vi "Set Window Topmost--lvapt.vi"(6 "Topmost(T)/Normal(F)":bool=TRUE, 8 "error in (no error)":errorcluster) -> (0 "error out":errorcluster)   [LabVIEW 2019]
uses:
  de497024-60f2-4a57-aa28-fde8f66e810e.vi
  WINUTIL.LLB/WINUTIL.lvlib
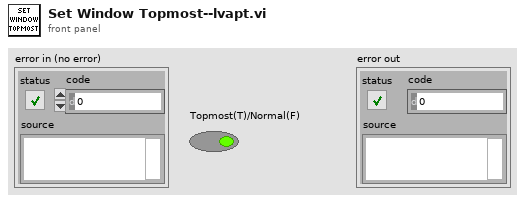
[diagram p1: front panel]
types:
  T1 = typedef "WINUTIL.lvlib/Window Refnum" = refnum<k1>
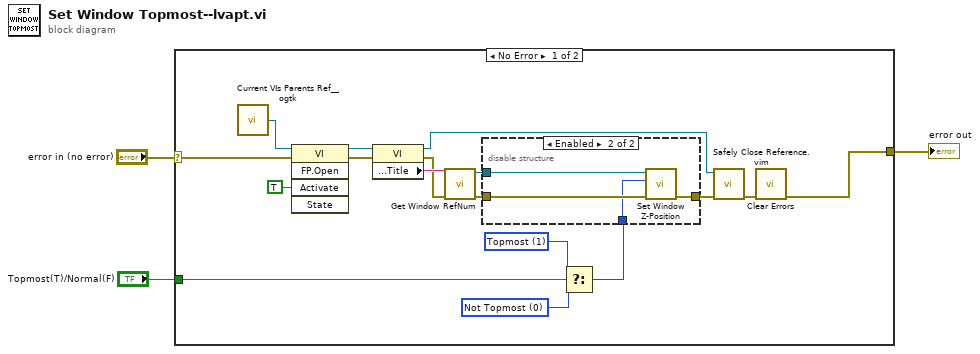
[diagram p0: block diagram]
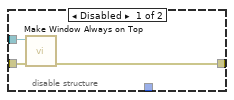
[diagram p2: hidden frame]
diagram:
  n1 = case shown="No Error" "error in (no error)" {
    selector: "error in (no error)" -> [w20 w28]
    tunnel: [w12 w28] -> w2
    tunnel: "Topmost(T)/Normal(F)" -> [w7 _]
    frame No Error {
      w5 = i16 0 items=["Not Topmost", "Topmost", "Top", "Bottom"] ("z-order position")
      w6 = i16 1 items=["Not Topmost", "Topmost", "Top", "Bottom"] ("z-order position")
      n2 = call <userlib>:"Current VIs Parents Ref__ogtk.vi"() -> ("Calling VI's Reference"=w11:refnum<vi>)  [unwired: 2 in]
      n3 = invoke class="VI" method="FP.Open"(reference=w11, error in=w20, "Activate"=TRUE ("Activate?")) -> (reference out=w17:refnum<vi>, error out=w18:errorcluster)  [unwired: 2 in, 3 out]
      n4 = property class="VI"(reference=w17, error in=w18) -> (reference out=w8:refnum<vi>, error out=w10:errorcluster, "Front Panel.Title"=w14:string)
      n5 = call "Get Window RefNum.vi"("error in (no error)"=w10, "window name (\"\")"=w14) -> ("error out"=w16:errorcluster, "window refnum (NaWR)"=w13:T1)  [unwired: 6 in]
      n6 = Select(t=w6, s=w7, f=w5) -> (s? t:f=w4:i16)
      n7 = disable-structure shown="Enabled" {
        disable-tunnel: w13 -> [w23 w25]
        disable-tunnel: [w22 w26] -> w15
        disable-tunnel: w16 -> [w21 w27]
        disable-tunnel: w4 -> [_ w24]
        frame Disabled {
          n8 = call "Make Window Always on Top.vi"("error in (no error)"=w21, "window refnum (NaWR)"=w23) -> ("error out"=w22:errorcluster)  [unwired: 4 in, 1 out]
        }
        frame Enabled {
          n9 = call "Set Window Z-Position.vi"("error in (no error)"=w27, "z-order position"=w24, "window refnum"=w25) -> ("error out"=w26:errorcluster)  [unwired: 3 in, 1 out]
        }
      }
      n10 = call "Safely Close Reference.vim"("error in (no error)"=w15, "LVClassLibrary in"=w8) -> ("error out"=w9:errorcluster)  [unwired: 9 in]
      n11 = call <vilib>:"Clear Errors.vi"("error in (no error)"=w9) -> ("error out"=w12:errorcluster)  [unwired: 5 in, 1 out]
    }
    frame Error {
    }
  }
  "error out" <- w2
